vi "gfitsio-check-image-for-read.vi"(4 "lpixel":i32[](array[numeric]), 5 "inc":i32[](array[numeric]), 6 "fpixel":i32[](array[numeric]), 8 "error in (no error)":errorcluster, 11 "gfits refnum":T1) -> (0 "error out":errorcluster, 1 "lpixel out":i32[](array[numeric]), 3 "dup gfits refnum":T1)   [LabVIEW 2015]
uses:
  gfitsio-refnum.ctl
panel:
  # "If -1 is supplied for lpixel this VI returns the actual lpixel of the image."
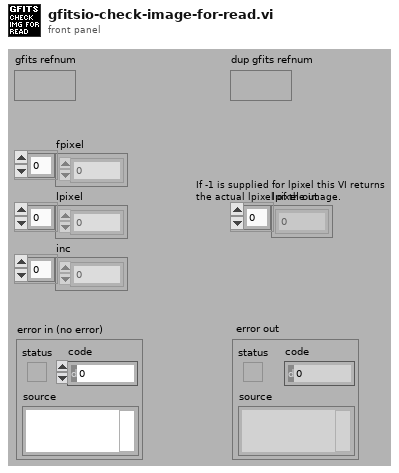
[diagram p1: front panel]
types:
  T1 = typedef "gfitsio-refnum.ctl" = refnum<k1>
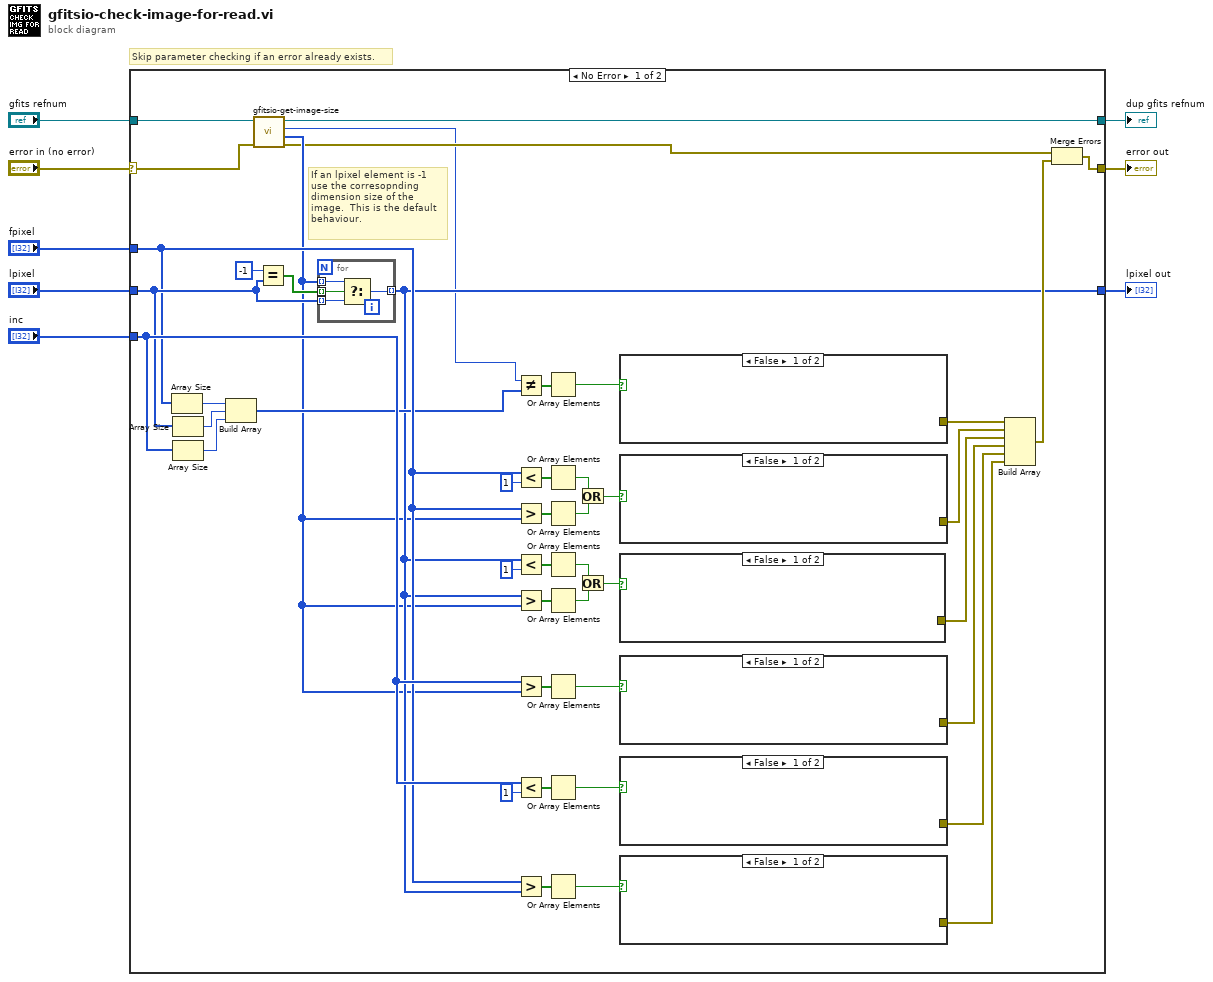
[diagram p0: block diagram]
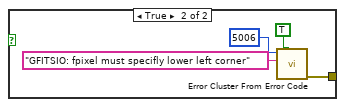
[diagram p2: hidden frame]
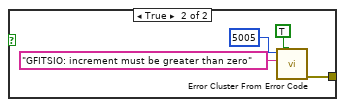
[diagram p3: hidden frame]
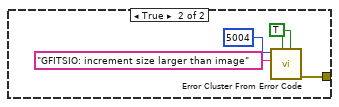
[diagram p4: hidden frame]
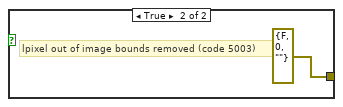
[diagram p5: hidden frame]
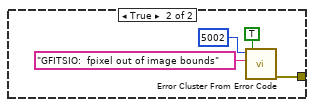
[diagram p6: hidden frame]
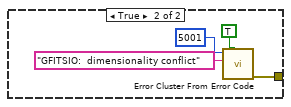
[diagram p7: hidden frame]
diagram:
  # "Skip parameter checking if an error already exists."
  n1 = case shown="No Error" "error in (no error)" {
    selector: "error in (no error)" -> [w52 w81]
    tunnel: "gfits refnum" -> [w53 w80]
    tunnel: [w10 w80] -> w3
    tunnel: "fpixel" -> [w20 _]
    tunnel: "lpixel" -> [w21 w79]
    tunnel: "inc" -> [w22 _]
    tunnel: [w51 w81] -> w8
    tunnel: [w13 w79] -> w1
    frame No Error {
      # "If an lpixel element is -1 use the corresopnding dimension size of the image.  This is the default behaviour."
      n2 = Array Size(array=w20) -> (size(s)=w19:i32)
      n3 = Array Size(array=w21) -> (size(s)=w18:i32)
      n4 = Array Size(array=w22) -> (size(s)=w17:i32)
      n5 = Build Array(w19, w18, w17) -> (w16:i32[])
      n6 = call "gfitsio-get-image-size.vi"("error in (no error)"=w52, "gfits refnum"=w53) -> ("error out"=w11:errorcluster, "naxes"=w12:i32[], "naxis"=w9:i32, "dup gfits refnum"=w10:T1)  [unwired: 6 in]
      n7 = Equal?(x=-1, y=w21) -> (x = y?=w23:bool[])
      n8 = for {
        tunnel: w12 -> [w56] mode=indexing
        tunnel: w23 -> [w55] mode=indexing
        tunnel: w21 -> [w57] mode=indexing
        tunnel: [w54] -> w13 mode=indexing
        n9 = Select(t=w56, s=w55, f=w57) -> (s? t:f=w54:i32)
      }
      n10 = Not Equal?(x=w9, y=w16) -> (x != y?=w15:bool[])
      n11 = Less?(x=w20, y=1 ("x")) -> (x < y?=w43:bool[])
      n12 = Greater?(x=w20, y=w12) -> (0:w42:bool[])
      n13 = Less?(x=w13, y=1 ("x")) -> (x < y?=w35:bool[])
      n14 = Greater?(x=w13, y=w12) -> (0:w36:bool[])
      n15 = Greater?(x=w22, y=w12) -> (0:w28:bool[])
      n16 = Less?(x=w22, y=1 ("x")) -> (x < y?=w30:bool[])
      n17 = Greater?(x=w20, y=w13) -> (0:w26:bool[])
      n18 = Or Array Elements(Boolean array=w15) -> (logical OR=w14:bool)
      n19 = Or Array Elements(Boolean array=w43) -> (logical OR=w40:bool)
      n20 = Or Array Elements(Boolean array=w42) -> (logical OR=w39:bool)
      n21 = Or Array Elements(Boolean array=w35) -> (logical OR=w37:bool)
      n22 = Or Array Elements(Boolean array=w36) -> (logical OR=w38:bool)
      n23 = Or Array Elements(Boolean array=w28) -> (logical OR=w27:bool)
      n24 = Or Array Elements(Boolean array=w30) -> (logical OR=w29:bool)
      n25 = Or Array Elements(Boolean array=w26) -> (logical OR=w25:bool)
      n26 = Or(x=w40, y=w39) -> (x .or. y?=w41:bool)
      n27 = Or(x=w37, y=w38) -> (x .or. y?=w33:bool)
      n28 = case shown="False" w14 {
        tunnel: [_ w76] -> w50
        frame False {
        }
        frame True {
          n29 = call <vilib>:"Error Cluster From Error Code.vi"("show call chain? (False)"=TRUE, "error message (\"\")"="GFITSIO:  dimensionality conflict" ("error message (\"\")"), "error code (0)"=5001) -> ("error out"=w76:errorcluster)  [unwired: 6 in]
        }
      }
      n30 = case shown="False" w41 {
        tunnel: [_ w72] -> w48
        frame False {
        }
        frame True {
          n31 = call <vilib>:"Error Cluster From Error Code.vi"("show call chain? (False)"=TRUE, "error message (\"\")"="GFITSIO:  fpixel out of image bounds" ("error message (\"\")"), "error code (0)"=5002) -> ("error out"=w72:errorcluster)  [unwired: 6 in]
        }
      }
      n32 = case shown="False" w33 {
        tunnel: [_ errorcluster {"status"=FALSE, "code"=0, "source"=""} ("error out")] -> w47
        frame False {
        }
        frame True {
          # "lpixel out of image bounds removed (code 5003)"
        }
      }
      n33 = case shown="False" w27 {
        tunnel: [_ w67] -> w46
        frame False {
        }
        frame True {
          w66 = TRUE ("show call chain? (False)")
          n34 = call <vilib>:"Error Cluster From Error Code.vi"("is warning? (False)"=w66, "show call chain? (False)"=w66, "error message (\"\")"="GFITSIO: increment size larger than image" ("error message (\"\")"), "error code (0)"=5004) -> ("error out"=w67:errorcluster)  [unwired: 5 in]
        }
      }
      n35 = case shown="False" w29 {
        tunnel: [_ w63] -> w45
        frame False {
        }
        frame True {
          n36 = call <vilib>:"Error Cluster From Error Code.vi"("show call chain? (False)"=TRUE, "error message (\"\")"="GFITSIO: increment must be greater than zero" ("error message (\"\")"), "error code (0)"=5005) -> ("error out"=w63:errorcluster)  [unwired: 6 in]
        }
      }
      n37 = case shown="False" w25 {
        tunnel: [_ w59] -> w32
        frame False {
        }
        frame True {
          n38 = call <vilib>:"Error Cluster From Error Code.vi"("show call chain? (False)"=TRUE, "error message (\"\")"="GFITSIO: fpixel must specifly lower left corner" ("error message (\"\")"), "error code (0)"=5006) -> ("error out"=w59:errorcluster)  [unwired: 6 in]
        }
      }
      n39 = Build Array(w50, w48, w47, w46, w45, w32) -> (w49:errorcluster[])
      n40 = Merge Errors(w11, w49) -> (w51:errorcluster)
    }
    frame Error {
    }
  }
  "error out" <- w8
  "dup gfits refnum" <- w3
  "lpixel out" <- w1
